vi "filter_static.vi"() -> ()   [LabVIEW 2017]
panel:
  out "Waveform Chart":dynamicdata(graph)
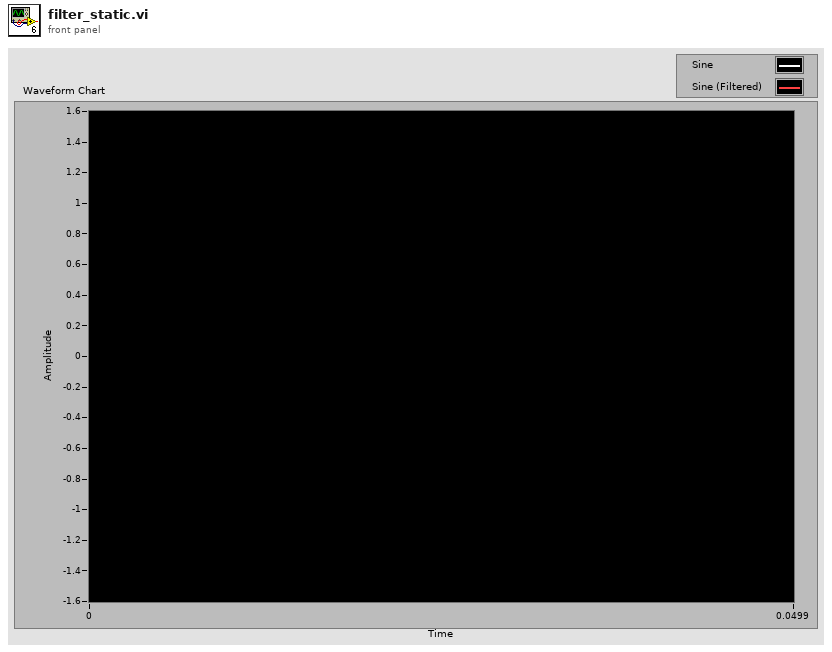
[diagram p1: front panel]
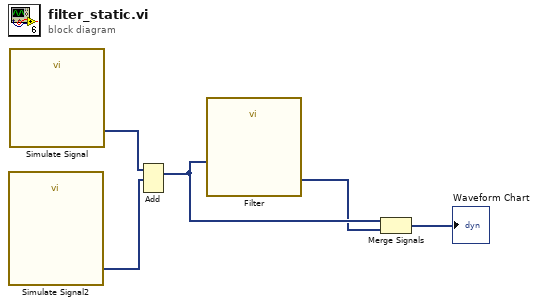
[diagram p0: block diagram]
diagram:
  n1 = call "Simulate Signal2"() -> ("Sine"=w3:dynamicdata)  [unwired: 14 in, 1 out]
  n2 = call "Simulate Signal"() -> ("Sine"=w2:dynamicdata)  [unwired: 14 in, 1 out]
  n3 = Add(1:w3, 2:w2) -> (0:w4:dynamicdata)  [unwired: 1 in, 1 out]
  n4 = call "Filter"("Signal"=w4) -> ("Filtered Signal"=w1:dynamicdata)  [unwired: 9 in, 1 out]
  n5 = Merge Signals(w4, w1) -> (→"Waveform Chart":dynamicdata)
